vi "LucaStopAcquisition.vi"(8 "error in (no error)":errorcluster) -> (0 "error out":errorcluster)   [LabVIEW 2009]
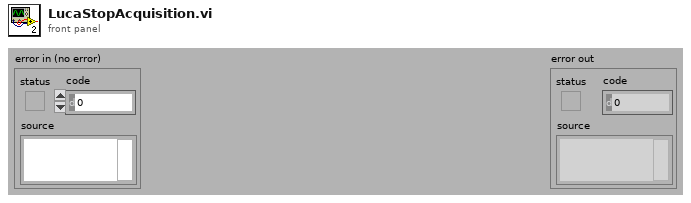
[diagram p1: front panel]
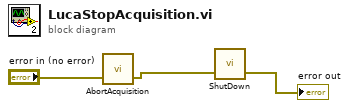
[diagram p0: block diagram]
diagram:
  n1 = call <userlib>:"AbortAcquisition.vi"("error in (no error)"="error in (no error)") -> ("error out"=w2:errorcluster)  [unwired: 1 in, 1 out]
  n2 = call <userlib>:"ShutDown.vi"("error in (no error)"=w2) -> ("error out"=→"error out":errorcluster)  [unwired: 1 in, 1 out]
